vi "Scale um To mm.vi"(11 "um":dbl) -> (3 "mm":dbl)   [LabVIEW 2015, in "Utility.lvlib"]
uses:
  Utility.lvlib
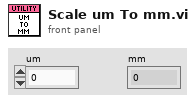
[diagram p1: front panel]
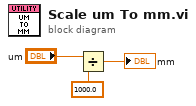
[diagram p0: block diagram]
diagram:
  n1 = Divide(x="um", y=1000.0) -> (x/y=→"mm":dbl)
